vi "LED Immediate.vi"(6 "Operation":T1, 7 "Description":string, 8 "Command Info In":T4, 9 "Amp or Speaker":T2, 10 "Lights State":T3, 11 "Match Time":dbl) -> (0 "Command Info Out":T4)   [LabVIEW 2023]
doc: "This template is useful for immediate subsystem actions that do not need deadband filtering\n\nBe sure to right-click and select New from Template and save with a new command name."
uses:
  <vilib>/Rock Robotics/WPI/Framework/Command Status Info.ctl
  <vilib>/Rock Robotics/WPI/Framework/Completion Status.ctl
  <vilib>/Rock Robotics/WPI/Framework/Completion Notifier.ctl
  source files/Amp-Speaker.ctl
  source files/Lights Setpoints.ctl
  Implementation/LED Operations.ctl
  Implementation/LED Setpoints.ctl
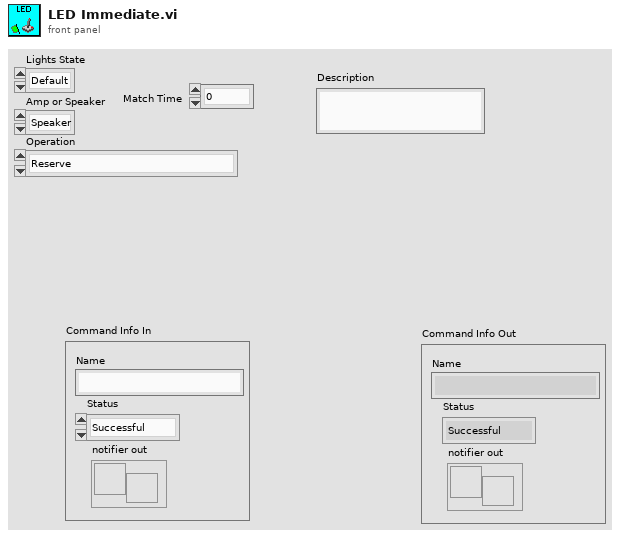
[diagram p1: front panel]
types:
  T1 = typedef "LED Operations.ctl" = enum16{"Reserve", "Read Current", "Immediate"}
  T2 = typedef "Lights Setpoints.ctl" = enum16{"Speaker", "Amp"}
  T3 = typedef "Amp-Speaker.ctl" = enum16{"Default", "Flywheel State", "Endgame", "Note Detection"}
  T4 = typedef "Command Status Info.ctl" = cluster{"Name":string, "Status":T5, "notifier out":T6}
  T5 = typedef "Completion Status.ctl" = enum16{"Successful", "Aborted", "Incomplete"}
  T6 = typedef "Completion Notifier.ctl" = refnum<notifier>
  T7 = typedef "LED Setpoints.ctl" = cluster{"Operation":T1, "Match Time":dbl, "Lights State":T3, "Amp or Speaker":T2}
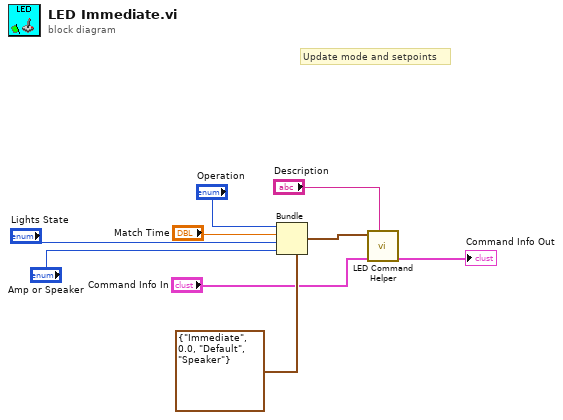
[diagram p0: block diagram]
diagram:
  # "Update mode and setpoints"
  n1 = Bundle(cluster=T7 {"Operation"=enum."Immediate", "Match Time"=0.0, "Lights State"=enum."Default", "Amp or Speaker"=enum."Speaker"} ("SubSystem Data"), "Operation"="Operation", "Match Time"="Match Time", "Lights State"="Lights State", "Amp or Speaker"="Amp or Speaker") -> (w5:T7)
  n2 = call "LED Command Helper.vi"("Description"="Description", "Command Info In"="Command Info In", "SubSystem Data"=w5) -> ("Command Info Out"=→"Command Info Out":T4)  [unwired: 6 in, 2 out]
